vi "Close.vi"(8 "error in":errorcluster, 11 "CanHandleIn":T1) -> (0 "error out":errorcluster, 3 "CanHandleOut":T1)   [LabVIEW 2011, in "Konvolucio MCAN120803.lvlib"]
doc: "Closes the CAN connection, sets the IsOpen property to false, and disposes of the internal Stream object."
uses:
  <instrlib>/Konvolucio MCAN120803/Konvolucio MCAN120803.lvlib
  <instrlib>/Konvolucio MCAN120803/Types/CanHandleType.ctl
  C:/Program Files/National Instruments/LabVIEW 2011/instr.lib/Konvolucio MCAN120803/Private/Konvolucio.MCAN120803.API.dll
  Private/Konvolucio.MCAN120803.API.dll
  <instrlib>/Konvolucio MCAN120803/Public/Attributes/AttrGetIsConnected.vi
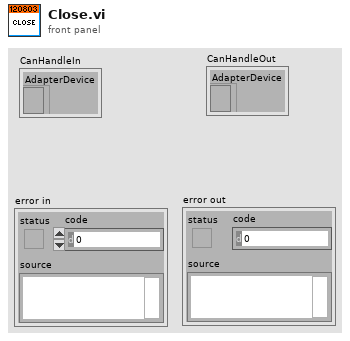
[diagram p1: front panel]
types:
  T1 = typedef "Konvolucio MCAN120803.lvlib/CanHandleType.ctl" = cluster{"AdapterDevice":refnum<k24>}
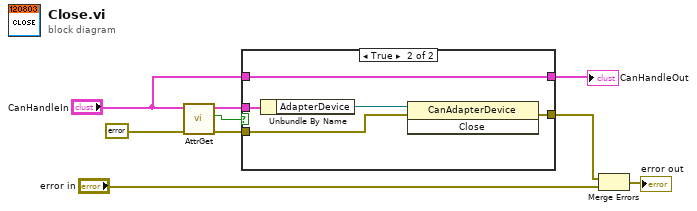
[diagram p0: block diagram]
diagram:
  n1 = call-poly <instrlib>:"AttrGet.vi"("error in"=errorcluster {"status"=FALSE, "code"=0, "source"=""}, "CanHandleIn"="CanHandleIn") -> ("error out"=w8:errorcluster, "State"=w7:bool, "CanHandleOut"=w9:T1)  [unwired: 7 in]
  n2 = case shown="True" w7 {
    tunnel: [w11 w16] -> w2
    tunnel: w9 -> [_ w14]
    tunnel: w8 -> [w11 w13]
    tunnel: "CanHandleIn" -> [w10 w12]
    tunnel: [w10 w12] -> w5
    frame False {
    }
    frame True {
      n3 = Unbundle By Name(w14) -> ("AdapterDevice"=w15:refnum<k24>)
      n4 = invoke class="CanAdapterDevice" method="Close"(reference=w15, error in=w13) -> (error out=w16:errorcluster)  [unwired: 1 in, 2 out]
    }
  }
  "CanHandleOut" <- w5
  n5 = Merge Errors(w2, "error in") -> (→"error out":errorcluster)
